vi "ToTable.vi"(8 "error in (no error)":errorcluster, 9 "Numeric":i32, 10 "variant":variant, 11 "node in":refnum<class "Modbus Module editor node.lvclass">) -> (0 "error out":errorcluster, 1 "row header":string[](array[string]), 2 "table":string[][](array[string]), 3 "node in out":refnum<class "Modbus Module editor node.lvclass">)   [LabVIEW 2015, in "Modbus Module editor node.lvclass"]
doc: "Copyright 2015 National Instruments Corporation\n\nLicensed under the Apache License, Version 2.0 (the \"License\"); you may not use this file except in compliance with the License. You may obtain a copy of the License at http://www.apache.org/licenses/LICENSE-2.0\nUnless required by applicable law or agreed to in writing, software distributed under the License is distributed on an \"AS IS\" BASIS, WITHOUT WARRANTIES OR CONDITIONS OF ANY KIND, either express or implied. See the License for the specific language governing permissions and limitations under the License."
uses:
  Modbus Module editor node.lvclass
  module/configuration/Modbus Module configuration.lvclass
  <vilib>/NI/Module Execution Interface/Engine Configuration/engine configuration.lvclass
  <vilib>/NI/Configuration Framework/serializable configuration/NISE_CEF_serializable configuration.lvclass/NISE_CEF_serializable configuration.ctl
  module/configuration/Modbus Module configuration.lvclass/Modbus Module configuration.ctl
  <vilib>/NI/Tag Bus/tag/tag descriptor.lvclass/tag descriptor.ctl
  <vilib>/NI/Tag Bus Module Framework/channel/TBM channel.lvclass/TBM channel.ctl
  <vilib>/NI/Tag Bus/tag/read tag name.vi
  <vilib>/NI/Tag Bus Module Framework/channel/Read channel classification.vi
  <vilib>/NI/Tag Bus/tag/read data type.vi
  <vilib>/NI/Configuration Framework/serializable configuration/Read UID.vi
  module/configuration/Read modbus channels.vi
  <vilib>/Utility/LVClass/Get LV Class Name.vi
  <vilib>/NI/Configuration Framework/error generator/NISE_error generator.vi
  module/module channel/Modbus Module Channel.lvclass
  <vilib>/NI/Tag Bus/tag/tag descriptor.lvclass
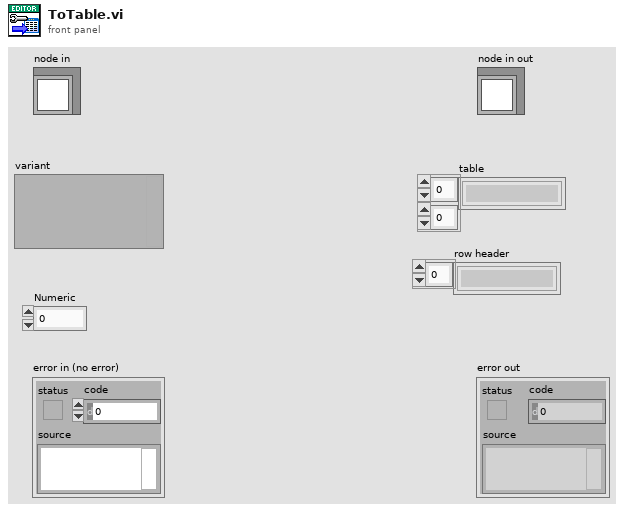
[diagram p1: front panel]
types:
  T1 = typedef "TBM channel.lvclass/channel classification.ctl" = enum16{"input data", "output data", "processing parameter", "processing result"}
  T2 = typedef "tag bus.lvlib/tag descriptor.lvclass/Data Type.ctl" = enum16{"Double", "Single", "I64", "I32", "I16", "I8", "U64", "U32", "U16", "U8", "Boolean", "String", "Array of Double", "Array of Single", "Array of I64", "Array of I32", "Array of I16", "Array of I8", "Array of U64", "Array of U32", "Array of U16", "Array of U8", "Array of Boolean", "Array of String"}
  T3 = typedef "Modbus Module editor node.lvclass/permissions.ctl" = enum32{"Read from MB", "Write to MB"}
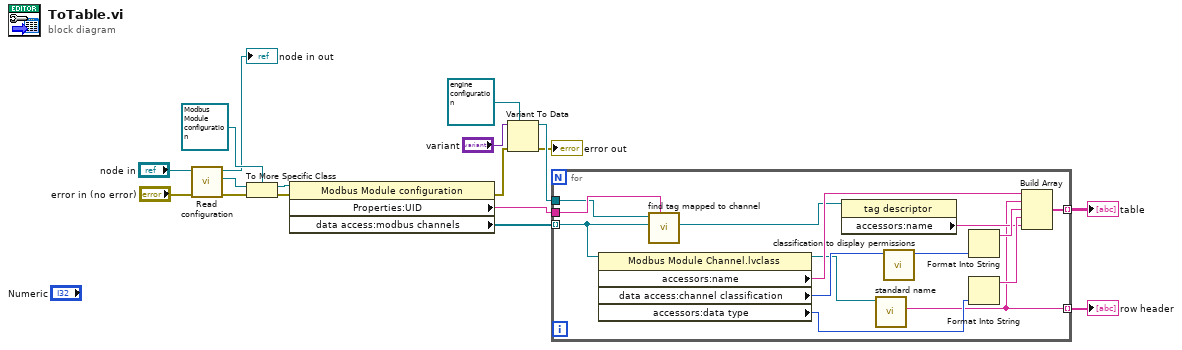
[diagram p0: block diagram]
diagram:
  n1 = call-dynamic "Read configuration.vi"("error in"="error in (no error)", "Modbus Slave editor node in"="node in") -> ("error out"=w4:errorcluster, "configuration"=w16:refnum<class "NISE_CEF_serializable configuration.lvclass">, "Modbus Slave editor node out"=→"node in out":refnum<class "Modbus Module editor node.lvclass">)  [unwired: 7 in]
  n2 = To More Specific Class(target class=refnum<class "Modbus Module configuration.lvclass"> refnum ("reference"), reference=w16, error in=w4) -> (specific class reference=w14:refnum<class "Modbus Module configuration.lvclass">, error out=w3:errorcluster)
  n3 = property class="Modbus Module configuration"(reference=w14, error in=w3) -> (error out=w1:errorcluster, "Properties:UID"=w12:string, "data access:modbus channels"=w13:refnum<class "Modbus Module Channel.lvclass">[])  [unwired: 1 out]
  n4 = Variant To Data(error in=w1, type=refnum<class "engine configuration.lvclass"> refnum ("engine configuration in"), Variant="variant") -> (data=w8:refnum<class "engine configuration.lvclass">, error out=→"error out":errorcluster)
  n5 = for {
    tunnel: w13 -> [w22] mode=indexing
    tunnel: w12 -> [w23]
    tunnel: [w20] -> w11 mode=indexing
    tunnel: w8 -> [w19]
    tunnel: [w18] -> w7 mode=indexing
    n6 = property class="Modbus Module Channel.lvclass"(reference=w22) -> (reference out=w25:refnum<class "Modbus Module Channel.lvclass">, "accessors:name"=w27:string, "data access:channel classification"=w28:T1, "accessors:data type"=w26:T2)  [unwired: 1 in, 1 out]
    n7 = call <vilib>:"find tag mapped to channel.vi"("owner"=w23, "channel"=w22, "engine configuration in"=w19) -> ("tag"=w24:refnum<class "tag descriptor.lvclass">)  [unwired: 6 in, 2 out]
    n8 = property class="tag descriptor"(reference=w24) -> ("accessors:name"=w21:string)  [unwired: 1 in, 2 out]
    n9 = call "standard name.vi"("Modbus Module Channel in"=w25) -> ("standard name"=w18:string)  [unwired: 8 in, 2 out]
    n10 = call "classification to display permissions.vi"("channel classification"=w28) -> ("permissions"=w30:T3)  [unwired: 10 in]
    n11 = Format Into String(w30) -> (resulting string=w29:string)  [unwired: 3 in, 1 out]
    n12 = Format Into String(w26) -> (resulting string=w31:string)  [unwired: 3 in, 1 out]
    n13 = Build Array(w27, w18, w29, w31, w21) -> (w20:string[])
  }
  "table" <- w11
  "row header" <- w7
